vi "Configure Ratio.vi"(0 "VISA resource name":refnum<visa-resource-name>, 5 "error in (no error)":errorcluster, 9 "Range":dbl, 11 "Resolution":dbl) -> (14 "VISA resource name out":refnum<visa-resource-name>, 19 "error out":errorcluster)   [LabVIEW 2020, in "Keithley 2100 Series.lvlib"]
doc: "Definition:\nThis function calculates the ratio of an input DC voltage to a reference DC voltage according to the following equation:\n\n Ratio = DC Input Voltage/ DC Reference Voltage\n\nRemote Interface Operation:\n\nUse the following command to make a RATIO measurement.\n\nCONFigure:VOLTage:DC:RATio {<range>|MIN|MAX|DEF},{<resolution>|MIN|MAX|DEF}"
uses:
  Keithley 2100 Series.lvlib
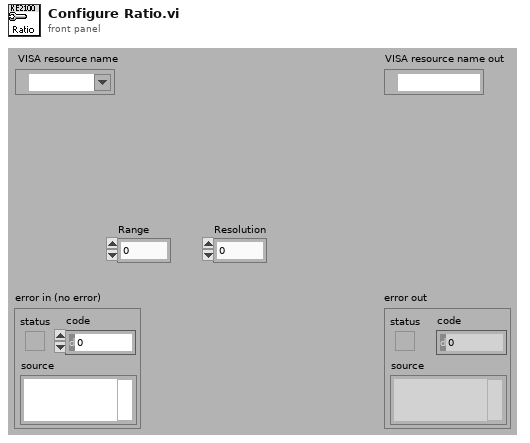
[diagram p1: front panel]
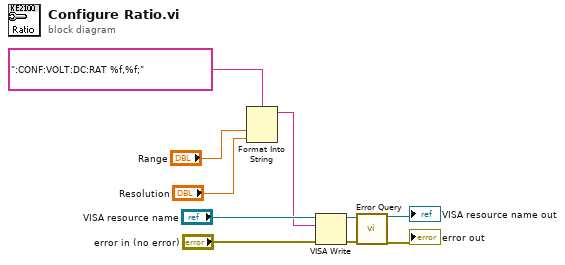
[diagram p0: block diagram]
diagram:
  n1 = Format Into String(format string=":CONF:VOLT:DC:RAT %f,%f;", "Range", "Resolution") -> (resulting string=w6:string)  [unwired: 2 in, 1 out]
  n2 = VISA Write(VISA resource name="VISA resource name", write buffer=w6, error in (no error)="error in (no error)") -> (VISA resource name out=w9:refnum<visa-resource-name>, error out=w10:errorcluster)  [unwired: 1 out]
  n3 = call "Error Query.vi"("VISA resource name"=w9, "error in (no error)"=w10) -> ("VISA resource name out"=→"VISA resource name out":refnum<visa-resource-name>, "error out"=→"error out":errorcluster)  [unwired: 14 in, 2 out]
